vi "Set and Get Active Row BG Color.vi"(6 "Active Row":i32, 7 "Mode":T1, 8 "错误输入":errorcluster, 10 "CellBG In":u32(colorbox), 11 "Listbox Ref":refnum<vi>) -> (0 "错误输出":errorcluster, 2 "CellBG Out":u32(colorbox), 3 "Dup Listbox Ref":refnum<vi>)   [LabVIEW 2012, in "Listbox Tool.lvlib"]
uses:
  Listbox Tool.lvlib
  Custom Type/Read and Write Mode.ctl
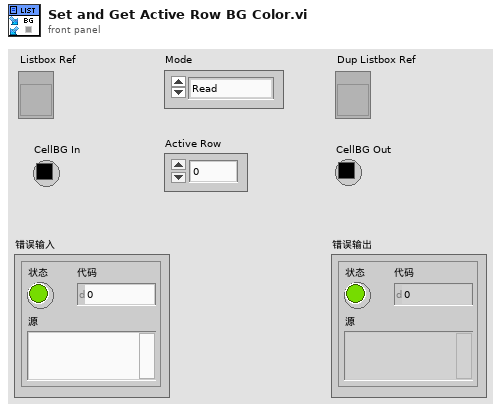
[diagram p1: front panel]
types:
  T1 = typedef "Listbox Tool.lvlib/Read and Write Mode.ctl" = enum16{"Read", "Write"}
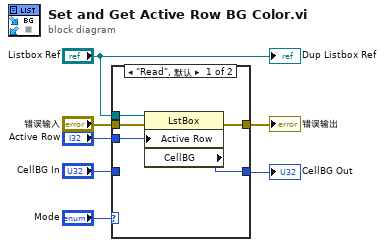
[diagram p0: block diagram]
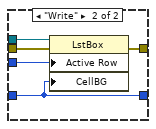
[diagram p2: hidden frame]
diagram:
  n1 = case shown="\"Read\", 默认" "Mode" {
    tunnel: "Listbox Ref" -> [w9 w13]
    tunnel: "Active Row" -> [w12 w17]
    tunnel: [w11 w16] -> w4
    tunnel: "CellBG In" -> [_ w16]
    tunnel: "错误输入" -> [w10 w15]
    tunnel: [w8 w14] -> w1
    frame "Read", Default {
      n2 = property class="LstBox"(reference=w9, error in=w10, "Active Row"=w12) -> (error out=w8:errorcluster, "CellBG"=w11:u32)  [unwired: 1 out]
    }
    frame "Write" {
      n3 = property class="LstBox"(reference=w13, error in=w15, "Active Row"=w17, "CellBG"=w16) -> (error out=w14:errorcluster)  [unwired: 1 out]
    }
  }
  "错误输出" <- w1
  "CellBG Out" <- w4
  "Dup Listbox Ref" <- "Listbox Ref"
